vi "Number to boolean cluster.vi"(1 "Numeric":u32) -> (0 "Output Channel Enable 2":T1)   [LabVIEW 2012]
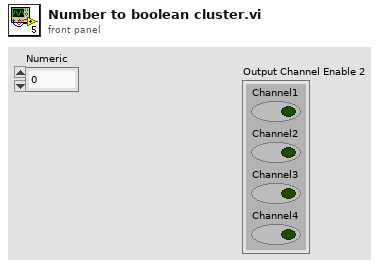
[diagram p1: front panel]
types:
  T1 = cluster{"Channel1":bool, "Channel2":bool, "Channel3":bool, "Channel4":bool}
  T2 = cluster{"Boolean array[0]":bool, "Boolean array[1]":bool, "Boolean array[2]":bool, "Boolean array[3]":bool, "Boolean array[4]":bool, "Boolean array[5]":bool, "Boolean array[6]":bool, "Boolean array[7]":bool, "Boolean array[8]":bool}
  T3 = cluster{"Boolean array[0]":bool, "Boolean array[1]":bool, "Boolean array[2]":bool, "Boolean array[3]":bool}
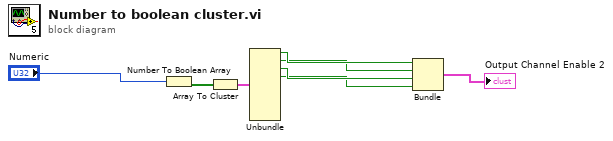
[diagram p0: block diagram]
diagram:
  n1 = Number To Boolean Array(number="Numeric") -> (Boolean array=w7:bool[])
  n2 = Array To Cluster(array=w7) -> (cluster=w6:T2)
  n3 = Unbundle(w6) -> ("Boolean array[0]"=w4:bool, "Boolean array[1]"=w3:bool, "Boolean array[2]"=w2:bool, "Boolean array[3]"=w1:bool)  [unwired: 5 out]
  n4 = Bundle("Boolean array[0]"=w4, "Boolean array[1]"=w3, "Boolean array[2]"=w2, "Boolean array[3]"=w1) -> (→"Output Channel Enable 2":T3)  [unwired: 1 in]
